vi "Autonomous Independent.vi"() -> ()   [LabVIEW 2013]
doc: "This VI is called when autonomous begins, and will automatically be terminated when autonomous ends. You can carry out timed or sensor driven robot movement independently without needing to return to the caller."
uses:
  AutoStates.ctl
  DoubleSolenoidAction.ctl
  ServoAction.ctl
  CollectorAction.ctl
  CollectorWrapAction.ctl
  TankDriveAction.ctl
  SonarAction.ctl
  AutoAlignMode.ctl
  ShooterWrapperAction.ctl
  Robot Global Data.vi
panel:
  in  "ServoInitAngle":i32=140
  in  "RaiseServoAngle":i32=100
  in  "PreShootWait":u32=500
  in  "MaxMotorChangeBackward":dbl=0.0025
  in  "PreRaiseArmWait":u32=500
  in  "MaxMotorChangeForward":dbl=0.05
  out "Drive3ftTimedOut?":bool
  out "CheckGoalTimedOut?":bool
  out "ElapsedTime":u32=7187
  out "StateTime":u32=1
  out "CurrentState":T1=enum."Stop"
  out "RaiseArmTimedOut":bool
  out "Hot?":bool
  out "Drive12ftTimedOut":bool
  out "LowerArmTimedOut":bool
  in  "CheckHotGoalTimeout":u32=1000
  in  "Drive3ftTimeout":u32
  in  "Drive3ftDistance":dbl=36.0 format="%#_13g"
  in  "RaiseArmTimeout":u32=800
  in  "Drive12ftDistance":dbl=150.0 format="%#_13g"
  in  "SlowdownDistance":dbl=24.0 format="%#_13g"
  in  "BrakeDistance":dbl=6.0 format="%#_13g"
  in  "Drive12ftTimeout":u32=4000
  in  "CollectorArmSpeed":dbl=1.0 format="%#_13g"
  in  "LiftArmWait":u32=200
  in  "DriveBackWait":u32
  in  "DriveBackSpeed":dbl
  in  "TwoBall?":bool
  in  "LowerArmTimeout":u32=800
  in  "error in":errorcluster
  out "error out":errorcluster
  # "ONE-BALL"
  # "GENERAL"
  # "TWO-BALL"
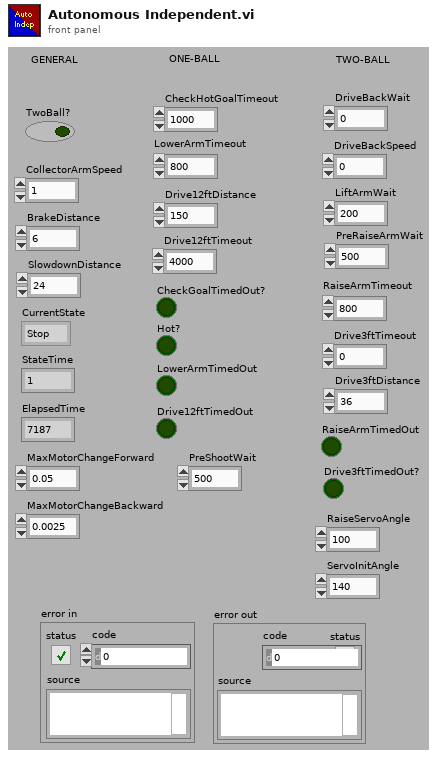
[diagram p1: front panel]
types:
  T1 = typedef "AutoStates.ctl" = enum16{"Init", "CheckHotGoal", "LowerArm", "PreCollect", "DriveBack", "Collect", "StopCollect", "LiftArm", "RaiseServo", "Drive12ft", "Shoot12ft", "RaiseArm", "Drive3ft", "Shoot3ft", "Stop"}
  T2 = typedef "DoubleSolenoidAction.ctl" = enum16{"Init", "Middle", "In", "Out"}
  T3 = typedef "ServoAction.ctl" = enum16{"Init", "SetAngle", "GetAngle", "Disable"}
  T4 = typedef "CollectorAction.ctl" = enum16{"Init", "Raise", "Lower", "Stop", "GetStatus"}
  T5 = typedef "CollectorWrapAction.ctl" = enum16{"PreCollect", "Collect", "Stop"}
  T6 = typedef "TankDriveAction.ctl" = enum16{"Init", "LinearDrive", "SetValue", "Disable"}
  T7 = typedef "AutoAlignMode.ctl" = enum16{"Fullspeed", "Linear"}
  T8 = typedef "SonarAction.ctl" = enum16{"Init", "ReadValue", "Disable"}
  T9 = typedef "ShooterWrapperAction.ctl" = enum16{"Init", "CollectorDown", "CollectorUp"}
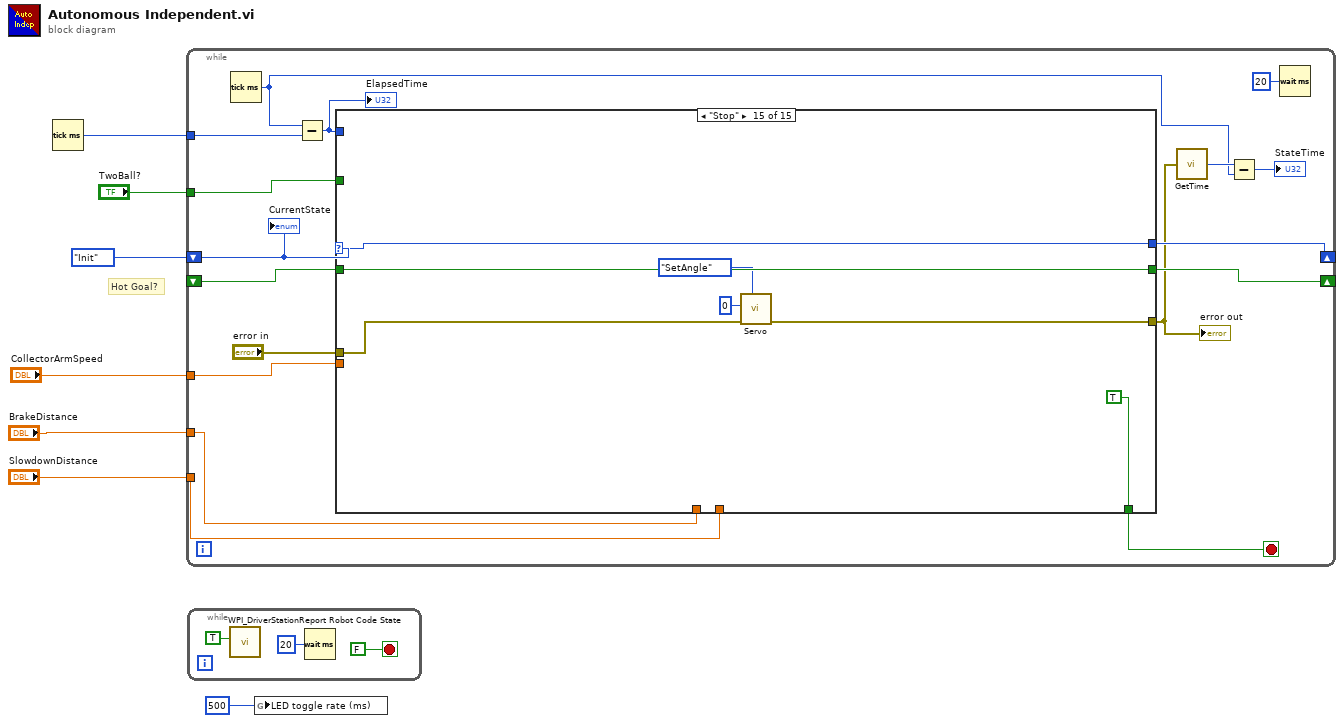
[diagram p0: block diagram]
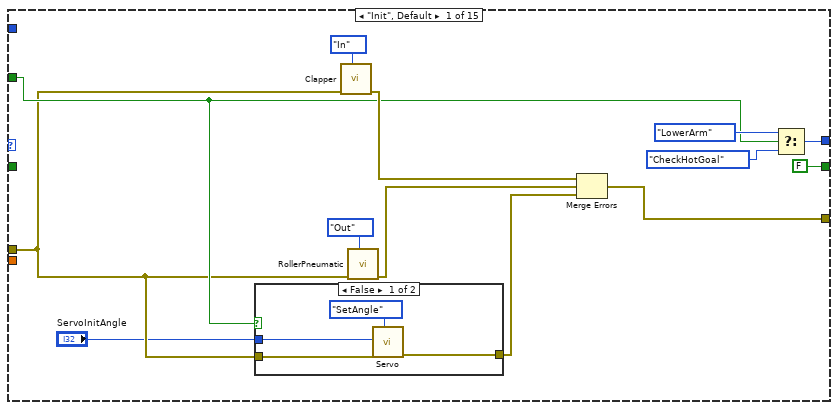
[diagram p2: hidden frame]
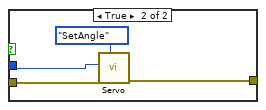
[diagram p3: hidden frame]
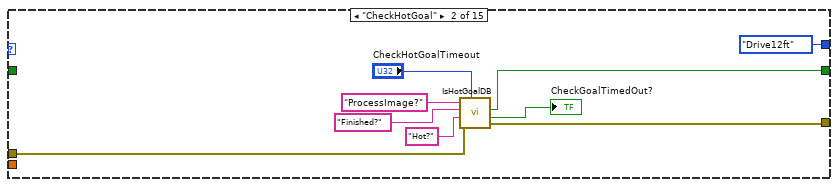
[diagram p4: hidden frame]
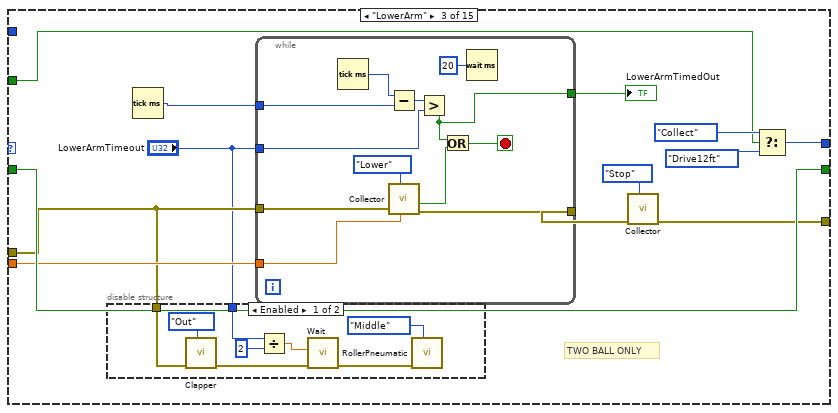
[diagram p5: hidden frame]
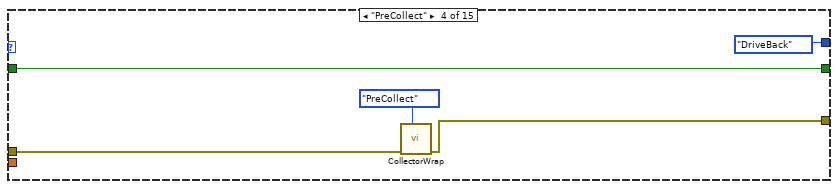
[diagram p7: hidden frame]
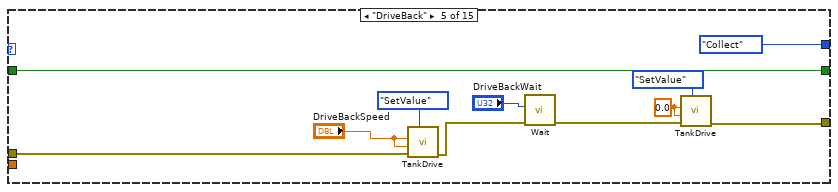
[diagram p8: hidden frame]
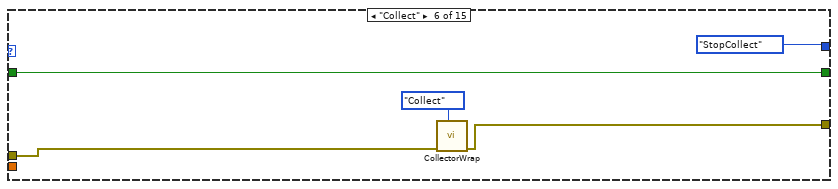
[diagram p9: hidden frame]
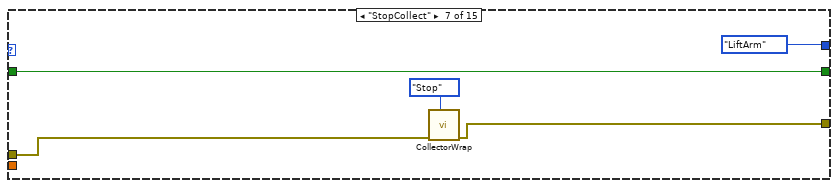
[diagram p10: hidden frame]
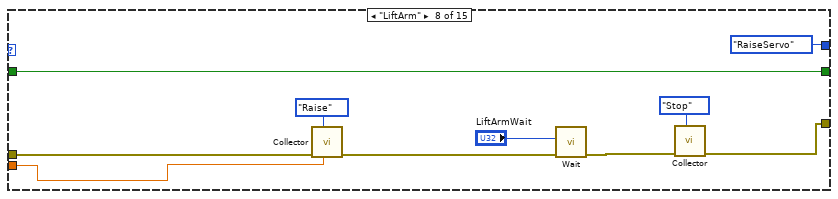
[diagram p11: hidden frame]
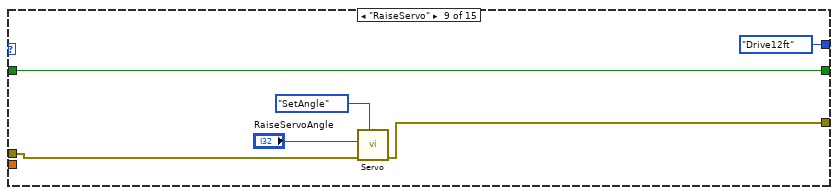
[diagram p12: hidden frame]
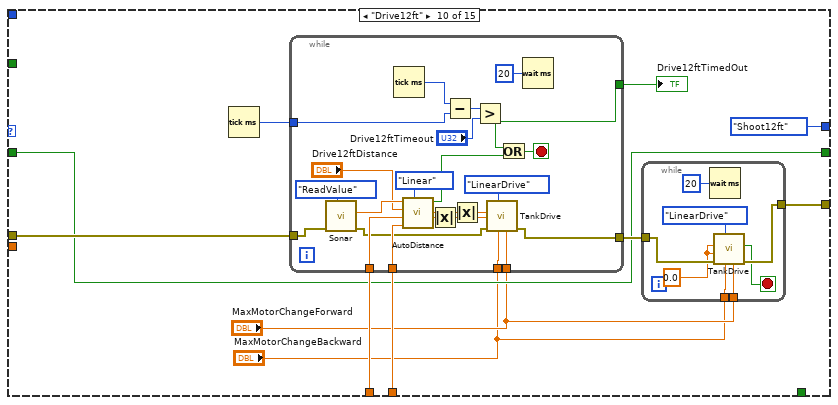
[diagram p13: hidden frame]
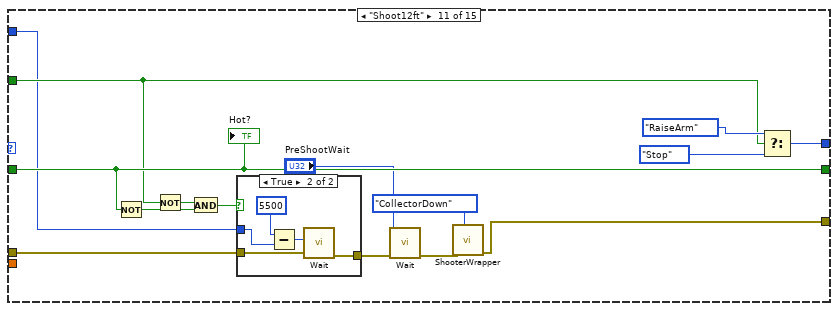
[diagram p14: hidden frame]
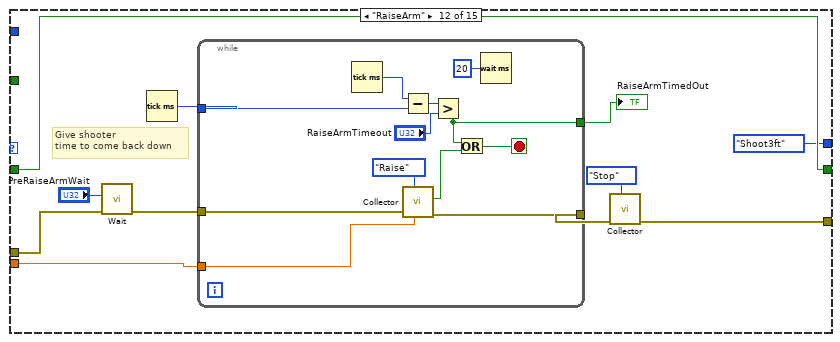
[diagram p16: hidden frame]
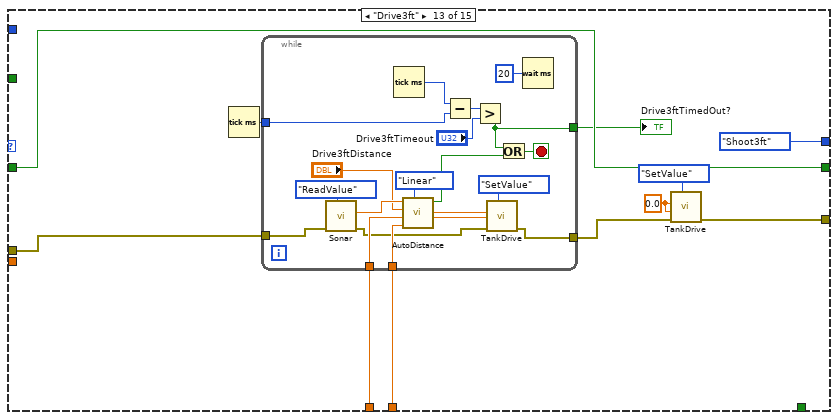
[diagram p17: hidden frame]
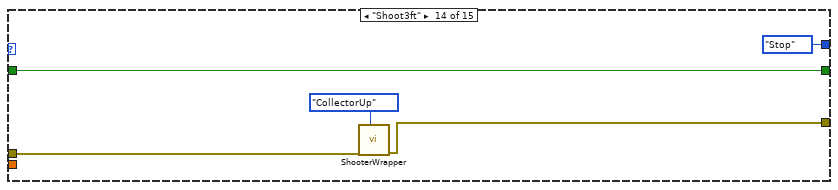
[diagram p18: hidden frame]
diagram:
  # "Hot Goal?"
  n1 = Tick Count (ms)() -> (millisecond timer value=w1:u32)
  n2 = while {
    shift-right: [w20] -> _
    shift-left: AutoStates."Init" ("Enum") -> [w24]
    shift-right: [w22] -> _
    shift-left: _ -> [w21]
    tunnel: "TwoBall?" -> [w19]
    tunnel: "CollectorArmSpeed" -> [w17]
    tunnel: "BrakeDistance" -> [w15]
    tunnel: "SlowdownDistance" -> [w16]
    tunnel: w1 -> [w14]
    stop <- w12 stop-if-true
    n3 = Tick Count (ms)() -> (millisecond timer value=w9:u32)
    n4 = Subtract(x=w9, y=w14) -> (x-y=w13:u32)
    "ElapsedTime" <- w13
    n5 = case shown="\"Stop\"" w24 {
      selector: w24 -> [_ _ _ _ _ _ _ _ _ _ _ _ _ _ w257]
      tunnel: "error in" -> [w27 w54 w56 w92 w103 w108 w113 w118 w128 w139 w182 w202 w224 w252 w258]
      tunnel: [w33 w53 w59 w91 w96 w107 w112 w117 w127 w133 w187 w198 w220 w251 w255] -> w11
      tunnel: [FALSE ("Hot?") w49 w66 w89 w101 w105 w110 w116 w129 w135 w180 w201 w222 w249 w259] -> w22
      tunnel: w21 -> [_ _ w66 w89 w101 w105 w110 w116 w129 w135 w180 w201 w222 w249 w259]
      tunnel: [w31 AutoStates."Drive12ft" ("Enum") w61 AutoStates."DriveBack" ("Enum") AutoStates."Collect" ("Enum") AutoStates."StopCollect" ("Enum") AutoStates."LiftArm" ("Enum") AutoStates."RaiseServo" ("Enum") AutoStates."Drive12ft" ("Enum") AutoStates."Shoot12ft" ("Enum") w183 AutoStates."Shoot3ft" ("Enum") AutoStates."Shoot3ft" ("Enum") AutoStates."Stop" ("Enum") w257] -> w20
      tunnel: w19 -> [w28 _ w62 _ _ _ _ _ _ _ w178 _ _ _ _]
      tunnel: w17 -> [_ _ w60 _ _ _ _ w115 _ _ _ w203 _ _ _]
      tunnel: w16 -> [_ _ _ _ _ _ _ _ _ w137 _ _ w225 _ _]
      tunnel: w15 -> [_ _ _ _ _ _ _ _ _ w136 _ _ w226 _ _]
      tunnel: w13 -> [_ _ _ _ _ _ _ _ _ _ w175 _ _ _ _]
      tunnel: [_ _ _ _ _ _ _ _ _ _ _ _ _ _ TRUE] -> w12
      frame "Init", Default {
        n6 = case shown="False" w28 {
          tunnel: w27 -> [w40 w45]
          tunnel: [w39 w44] -> w26
          tunnel: "ServoInitAngle" -> [w38 w42]
          frame False {
            n7 = call "Servo.vi"("Action"=ServoAction."SetAngle", "error in (no error)"=w40, "Angle (deg)"=w38) -> ("error out"=w39:errorcluster)  [unwired: 7 in, 1 out]
          }
          frame True {
            n8 = call "Servo.vi"("Action"=ServoAction."SetAngle", "error in (no error)"=w45, "Angle (deg)"=w42) -> ("error out"=w44:errorcluster)  [unwired: 7 in, 1 out]
          }
        }
        n9 = call "Clapper.vi"("State"=DoubleSolenoidAction."In", "Error in"=w27) -> ("Error out"=w35:errorcluster)  [unwired: 9 in]
        n10 = call "RollerPneumatic.vi"("State"=DoubleSolenoidAction."Out", "Error in"=w27) -> ("Error out"=w34:errorcluster)  [unwired: 9 in]
        n11 = Merge Errors(w35, w34, w26) -> (w33:errorcluster)
        n12 = Select(t=AutoStates."LowerArm" ("Enum"), s=w28, f=AutoStates."CheckHotGoal" ("Enum")) -> (s? t:f=w31:T1)
      }
      frame "CheckHotGoal" {
        n13 = call "IsHotGoalDB.vi"("Timeout (ms)"="CheckHotGoalTimeout", "error in"=w54, "DBHot?"="Hot?", "DBFinished?"="Finished?", "DBStart"="ProcessImage?") -> ("error out"=w53:errorcluster, "TimedOut?"=→"CheckGoalTimedOut?":bool, "Hot?"=w49:bool)  [unwired: 4 in]
      }
      frame "LowerArm" {
        # "TWO BALL ONLY"
        n14 = disable-structure shown="Enabled" {
          disable-tunnel: w56 -> [w75 _]
          disable-tunnel: "LowerArmTimeout" -> [w74 _]
          frame Enabled {
            n15 = call "Clapper.vi"("State"=DoubleSolenoidAction."Out", "Error in"=w75) -> ("Error out"=w71:errorcluster)  [unwired: 9 in]
            n16 = Divide(x=w74, y=u32 2) -> (x/y=w72:dbl)
            n17 = call "Wait.vi"("error in"=w71, "milliseconds to wait"=w72) -> ("error out"=w69:errorcluster)  [unwired: 9 in]
            n18 = call "RollerPneumatic.vi"("State"=DoubleSolenoidAction."Middle", "Error in"=w69) -> ()  [unwired: 9 in, 1 out]
          }
          frame Disabled {
          }
        }
        n19 = Tick Count (ms)() -> (millisecond timer value=w65:u32)
        n20 = while {
          tunnel: w56 -> [w87]
          tunnel: [w86] -> w67
          tunnel: w65 -> [w79]
          tunnel: w60 -> [w78]
          tunnel: [w77] -> w57
          tunnel: "LowerArmTimeout" -> [w76]
          stop <- w81 stop-if-true
          n21 = Tick Count (ms)() -> (millisecond timer value=w83:u32)
          n22 = Subtract(x=w83, y=w79) -> (x-y=w84:u32)
          n23 = call "Collector.vi"("MotorSpeed"=w78, "Action"=CollectorAction."Lower", "Error in"=w87) -> ("Error out"=w86:errorcluster, "Lower Triggered?"=w80:bool)  [unwired: 6 in, 1 out]
          n24 = Greater?(x=w84, y=w76) -> (0:w77:bool)
          n25 = Or(x=w77, y=w80) -> (x .or. y?=w81:bool)
          n26 = Wait (ms)(milliseconds to wait=u32 20) -> ()  [unwired: 1 out]
        }
        "LowerArmTimedOut" <- w57
        n27 = call "Collector.vi"("Action"=CollectorAction."Stop", "Error in"=w67) -> ("Error out"=w59:errorcluster)  [unwired: 7 in, 2 out]
        n28 = Select(t=AutoStates."Collect" ("Enum"), s=w62, f=AutoStates."Drive12ft" ("Enum")) -> (s? t:f=w61:T1)
      }
      frame "PreCollect" {
        n29 = call "CollectorWrap.vi"("Action"=CollectorWrapAction."PreCollect", "error in"=w92) -> ("error out"=w91:errorcluster)  [unwired: 9 in]
      }
      frame "DriveBack" {
        w94 = 0.0 ("LeftDesired")
        n30 = call "TankDrive.vi"("DriveAction"=TankDriveAction."SetValue", "error in (no error)"=w103, "RightDesired"="DriveBackSpeed", "LeftDesired"="DriveBackSpeed") -> ("error out"=w102:errorcluster)  [unwired: 6 in, 1 out]
        n31 = call "Wait.vi"("error in"=w102, "milliseconds to wait"="DriveBackWait") -> ("error out"=w97:errorcluster)  [unwired: 9 in]
        n32 = call "TankDrive.vi"("DriveAction"=TankDriveAction."SetValue", "error in (no error)"=w97, "RightDesired"=w94, "LeftDesired"=w94) -> ("error out"=w96:errorcluster)  [unwired: 6 in, 1 out]
      }
      frame "Collect" {
        n33 = call "CollectorWrap.vi"("Action"=CollectorWrapAction."Collect", "error in"=w108) -> ("error out"=w107:errorcluster)  [unwired: 9 in]
      }
      frame "StopCollect" {
        n34 = call "CollectorWrap.vi"("Action"=CollectorWrapAction."Stop", "error in"=w113) -> ("error out"=w112:errorcluster)  [unwired: 9 in]
      }
      frame "LiftArm" {
        n35 = call "Collector.vi"("MotorSpeed"=w115, "Action"=CollectorAction."Raise" ("CollectorAction"), "Error in"=w118) -> ("Error out"=w119:errorcluster)  [unwired: 6 in, 2 out]
        n36 = call "Wait.vi"("error in"=w119, "milliseconds to wait"="LiftArmWait") -> ("error out"=w120:errorcluster)  [unwired: 9 in]
        n37 = call "Collector.vi"("Action"=CollectorAction."Stop" ("CollectorAction"), "Error in"=w120) -> ("Error out"=w117:errorcluster)  [unwired: 7 in, 2 out]
      }
      frame "RaiseServo" {
        n38 = call "Servo.vi"("Action"=ServoAction."SetAngle", "error in (no error)"=w128, "Angle (deg)"="RaiseServoAngle") -> ("error out"=w127:errorcluster)  [unwired: 7 in, 1 out]
      }
      frame "Drive12ft" {
        n39 = Tick Count (ms)() -> (millisecond timer value=w140:u32)
        n40 = while {
          tunnel: w139 -> [w158]
          tunnel: [w162] -> w138
          tunnel: w140 -> [w167]
          tunnel: w137 -> [w160]
          tunnel: w136 -> [w161]
          tunnel: [w153] -> w132
          tunnel: "MaxMotorChangeForward" -> [w150]
          tunnel: "MaxMotorChangeBackward" -> [w149]
          stop <- w164 stop-if-true
          n41 = call "Sonar.vi"("Action"=SonarAction."ReadValue", "error in (no error)"=w158) -> ("error out"=w154:errorcluster, "distance"=w157:dbl)  [unwired: 8 in]
          n42 = Tick Count (ms)() -> (millisecond timer value=w168:u32)
          n43 = call "AutoDistance.vi"("Mode"=AutoAlignMode."Linear", "Slowdown"=w160, "Brake"=w161, "DesiredDistance"="Drive12ftDistance", "CurrentDistance"=w157) -> ("TankDriveRight"=w171:dbl, "TankDriveLeft"=w172:dbl, "Finished"=w163:bool)  [unwired: 4 in]
          n44 = Absolute Value(x=w171) -> (abs(x)=w151:dbl)
          n45 = Subtract(x=w168, y=w167) -> (x-y=w166:u32)
          n46 = Absolute Value(x=w172) -> (abs(x)=w152:dbl)
          n47 = Greater?(x=w166, y="Drive12ftTimeout") -> (0:w153:bool)
          n48 = call "TankDrive.vi"("MaxMotorChangeForward"=w150, "MaxMotorChangeBackwrad"=w149, "DriveAction"=TankDriveAction."LinearDrive", "error in (no error)"=w154, "RightDesired"=w151, "LeftDesired"=w152) -> ("error out"=w162:errorcluster)  [unwired: 4 in, 1 out]
          n49 = Or(x=w153, y=w163) -> (x .or. y?=w164:bool)
          n50 = Wait (ms)(milliseconds to wait=u32 20) -> ()  [unwired: 1 out]
        }
        "Drive12ftTimedOut" <- w132
        n51 = while {
          tunnel: w138 -> [w148]
          tunnel: [w147] -> w133
          tunnel: "MaxMotorChangeForward" -> [w142]
          tunnel: "MaxMotorChangeBackward" -> [w141]
          stop <- w143 stop-if-true
          w146 = 0.0 ("LeftDesired")
          n52 = Wait (ms)(milliseconds to wait=u32 20) -> ()  [unwired: 1 out]
          n53 = call "TankDrive.vi"("MaxMotorChangeForward"=w142, "MaxMotorChangeBackwrad"=w141, "DriveAction"=TankDriveAction."LinearDrive", "error in (no error)"=w148, "RightDesired"=w146, "LeftDesired"=w146) -> ("error out"=w147:errorcluster, "InRange?"=w143:bool)  [unwired: 4 in]
        }
      }
      frame "Shoot12ft" {
        n54 = Not(x=w180) -> (.not. x?=w176:bool)
        n55 = Not(x=w178) -> (.not. x?=w179:bool)
        n56 = And(x=w179, y=w176) -> (x .and. y?=w181:bool)
        n57 = case shown="True" w181 {
          tunnel: w182 -> [w188 w193]
          tunnel: [w188 w192] -> w177
          tunnel: w175 -> [_ w191]
          frame False {
          }
          frame True {
            n58 = Subtract(x=u32 5500 ("milliseconds to wait"), y=w191) -> (x-y=w189:u32)
            n59 = call "Wait.vi"("error in"=w193, "milliseconds to wait"=w189) -> ("error out"=w192:errorcluster)  [unwired: 9 in]
          }
        }
        n60 = call "Wait.vi"("error in"=w177, "milliseconds to wait"="PreShootWait") -> ("error out"=w174:errorcluster)  [unwired: 9 in]
        n61 = call "ShooterWrapper.vi"("Action"=ShooterWrapperAction."CollectorDown", "error in"=w174) -> ("error out"=w187:errorcluster)  [unwired: 8 in]
        n62 = Select(t=AutoStates."RaiseArm" ("Enum"), s=w178, f=AutoStates."Stop" ("Enum")) -> (s? t:f=w183:T1)
        "Hot?" <- w180
      }
      frame "RaiseArm" {
        # "Give shooter\ntime to come back down"
        n63 = call "Wait.vi"("error in"=w202, "milliseconds to wait"="PreRaiseArmWait") -> ("error out"=w195:errorcluster)  [unwired: 9 in]
        n64 = Tick Count (ms)() -> (millisecond timer value=w204:u32)
        n65 = while {
          tunnel: w195 -> [w216]
          tunnel: [w215] -> w200
          tunnel: w204 -> [w208]
          tunnel: w203 -> [w207]
          tunnel: [w206] -> w196
          stop <- w209 stop-if-true
          n66 = Tick Count (ms)() -> (millisecond timer value=w211:u32)
          n67 = Subtract(x=w211, y=w208) -> (x-y=w212:u32)
          n68 = call "Collector.vi"("MotorSpeed"=w207, "Action"=CollectorAction."Raise", "Error in"=w216) -> ("Error out"=w215:errorcluster, "Upper Triggered?"=w205:bool)  [unwired: 6 in, 1 out]
          n69 = Greater?(x=w212, y="RaiseArmTimeout") -> (0:w206:bool)
          n70 = Or(x=w206, y=w205) -> (x .or. y?=w209:bool)
          n71 = Wait (ms)(milliseconds to wait=u32 20) -> ()  [unwired: 1 out]
        }
        "RaiseArmTimedOut" <- w196
        n72 = call "Collector.vi"("Action"=CollectorAction."Stop", "Error in"=w200) -> ("Error out"=w198:errorcluster)  [unwired: 7 in, 2 out]
      }
      frame "Drive3ft" {
        w218 = 0.0 ("LeftDesired")
        n73 = Tick Count (ms)() -> (millisecond timer value=w227:u32)
        n74 = while {
          tunnel: w224 -> [w233]
          tunnel: [w237] -> w223
          tunnel: w227 -> [w242]
          tunnel: w225 -> [w235]
          tunnel: w226 -> [w236]
          tunnel: [w228] -> w217
          stop <- w239 stop-if-true
          n75 = call "Sonar.vi"("Action"=SonarAction."ReadValue", "error in (no error)"=w233) -> ("error out"=w229:errorcluster, "distance"=w232:dbl)  [unwired: 8 in]
          n76 = Tick Count (ms)() -> (millisecond timer value=w243:u32)
          n77 = call "AutoDistance.vi"("Mode"=AutoAlignMode."Linear", "Slowdown"=w235, "Brake"=w236, "DesiredDistance"="Drive3ftDistance", "CurrentDistance"=w232) -> ("TankDriveRight"=w246:dbl, "TankDriveLeft"=w247:dbl, "Finished"=w238:bool)  [unwired: 4 in]
          n78 = Subtract(x=w243, y=w242) -> (x-y=w241:u32)
          n79 = Greater?(x=w241, y="Drive3ftTimeout") -> (0:w228:bool)
          n80 = call "TankDrive.vi"("DriveAction"=TankDriveAction."SetValue", "error in (no error)"=w229, "RightDesired"=w246, "LeftDesired"=w247) -> ("error out"=w237:errorcluster)  [unwired: 6 in, 1 out]
          n81 = Or(x=w228, y=w238) -> (x .or. y?=w239:bool)
          n82 = Wait (ms)(milliseconds to wait=u32 20) -> ()  [unwired: 1 out]
        }
        "Drive3ftTimedOut?" <- w217
        n83 = call "TankDrive.vi"("DriveAction"=TankDriveAction."SetValue", "error in (no error)"=w223, "RightDesired"=w218, "LeftDesired"=w218) -> ("error out"=w220:errorcluster)  [unwired: 6 in, 1 out]
      }
      frame "Shoot3ft" {
        n84 = call "ShooterWrapper.vi"("Action"=ShooterWrapperAction."CollectorUp", "error in"=w252) -> ("error out"=w251:errorcluster)  [unwired: 8 in]
      }
      frame "Stop" {
        n85 = call "Servo.vi"("Action"=ServoAction."SetAngle", "error in (no error)"=w258, "Angle (deg)"=0) -> ("error out"=w255:errorcluster)  [unwired: 7 in, 1 out]
      }
    }
    "error out" <- w11
    n86 = call "GetTime.vi"("error in"=w11) -> ("Time"=w10:u32)
    n87 = Subtract(x=w10, y=w9) -> (x-y=→"StateTime":u32)
    n88 = Wait (ms)(milliseconds to wait=u32 20) -> ()  [unwired: 1 out]
    "CurrentState" <- w24
  }
  n89 = while {
    stop <- FALSE stop-if-true
    n90 = call <vilib>:"WPI_DriverStationReport Robot Code State.vi"("Autonomous"=TRUE) -> ()  [unwired: 10 in, 1 out]
    n91 = Wait (ms)(milliseconds to wait=u32 20) -> ()  [unwired: 1 out]
  }
  n92 = global write "Robot Global Data.vi" "LED toggle rate (ms)"(u32 500 ("LED ms toggle rate")) -> ()
